vi "GET_Origin.vi"(8 "error in (no error)":errorcluster, 11 "Layer.lvclass in":refnum<class "Layer.lvclass">) -> (0 "error out":errorcluster, 2 "Point32":T1, 3 "Layer.lvclass out":refnum<class "Layer.lvclass">)   [LabVIEW 2020, in "Layer.lvclass"]
doc: "Returns the Original coordinates of the User Layer."
uses:
  Layer.lvclass
  Layer.lvclass/Layer.ctl
  <vilib>/Utility/miscctls.llb/LVPoint32TypeDef.ctl
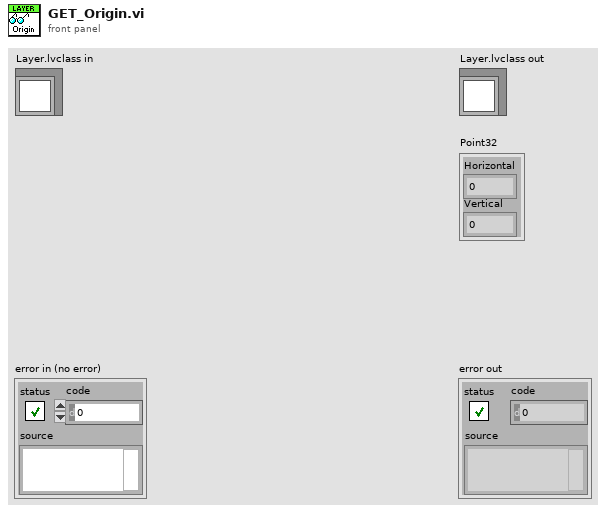
[diagram p1: front panel]
types:
  T1 = typedef "LVPoint32TypeDef.ctl" = cluster{"Horizontal":i32, "Vertical":i32}
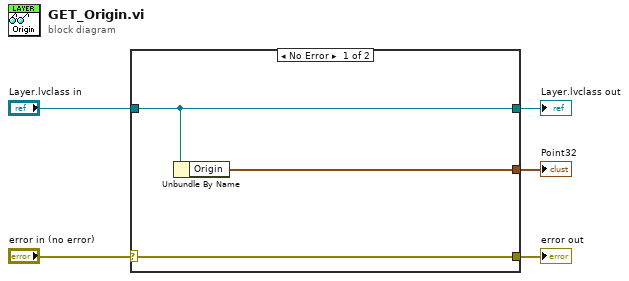
[diagram p0: block diagram]
diagram:
  n1 = case shown="No Error" "error in (no error)" {
    selector: "error in (no error)" -> [w8 w9]
    tunnel: [w8 w9] -> w4
    tunnel: [w7 w10] -> w2
    tunnel: "Layer.lvclass in" -> [w7 w10]
    tunnel: [w6 _] -> w1
    frame No Error {
      n2 = Unbundle By Name(w7) -> ("Origin"=w6:T1)
    }
    frame Error {
    }
  }
  "error out" <- w4
  "Layer.lvclass out" <- w2
  "Point32" <- w1
